vi "VMImport.vi"(8 "error in (no error)":errorcluster, 10 "VariableManager":refnum<class "VariableManager.lvclass">, 11 "VariableManagerRef in":refnum<vi>) -> (0 "error out":errorcluster, 3 "VariableManagerRef out":refnum<vi>)   [LabVIEW 2013, in "VariableManagerAPI.lvlib"]
doc: "Import the given VariableManager to overwrite the object in the reference.\nUpdateEvent and LastAcquireValues from original VariableManager will be transfered to the imported VariableManager."
uses:
  VariableManagerAPI.lvlib
  VariableManager/VariableManager.lvclass
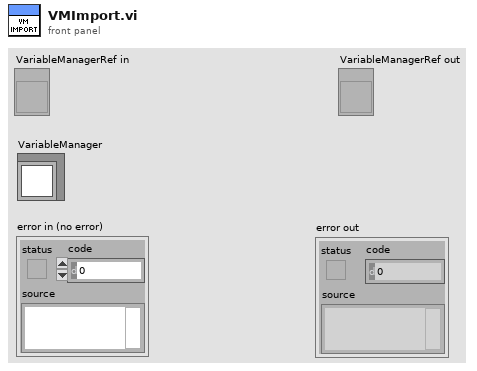
[diagram p1: front panel]
types:
  T1 = typedef "Semaphore RefNum" = refnum<k1>
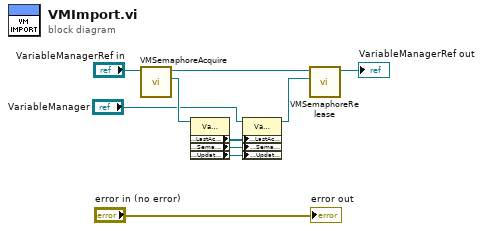
[diagram p0: block diagram]
diagram:
  n1 = call "VMSemaphoreAcquire.vi"("VariableManagerRef in"="VariableManagerRef in") -> ("VariableManager"=w7:refnum<class "VariableManager.lvclass">, "VariableManagerRef out"=w9:refnum<vi>)  [unwired: 7 in, 2 out]
  n2 = property class="VariableManager.lvclass"(reference=w7) -> ("Accessors:LastAcquireValues"=w5:refnum<class "VariableValue.lvclass">[], "Accessors:Semaphore"=w4:T1, "Accessors:UpdateEvent"=w3:refnum<user-event>)  [unwired: 1 in, 2 out]
  n3 = property class="VariableManager.lvclass"(reference="VariableManager", "Accessors:LastAcquireValues"=w5, "Accessors:Semaphore"=w4, "Accessors:UpdateEvent"=w3) -> (reference out=w2:refnum<class "VariableManager.lvclass">)  [unwired: 1 in, 1 out]
  n4 = call "VMSemaphoreRelease.vi"("VariableManager"=w2, "VariableManagerRef in"=w9) -> ("VariableManagerRef out"=→"VariableManagerRef out":refnum<vi>)  [unwired: 8 in, 1 out]
  "error out" <- "error in (no error)"
